vi "3_2_Circular convolution.vi"(4 "N-Point (auto/user def)":enum16{"AUTOMATIC", "USER DEFINED"}(ring), 5 "sequence h[n]":dbl[](array[numeric]), 6 "N-Point":dbl, 7 "sequence x[n]":dbl[](array[numeric])) -> (0 "Sequence y[n] = x[n] * h[n]":dbl[](graph), 1 "Sequence h[n]":dbl[](graph), 2 "Sequence x[n]":dbl[](graph), 3 "sequence y[n] = x[n] * h[n]":dbl[](array[numeric]))   [LabVIEW 2009]
panel:
  in  "stop":bool
  # "CIRCULAR CONVOLUTION"
  # "Program Developed by Indranil Sinharoy"
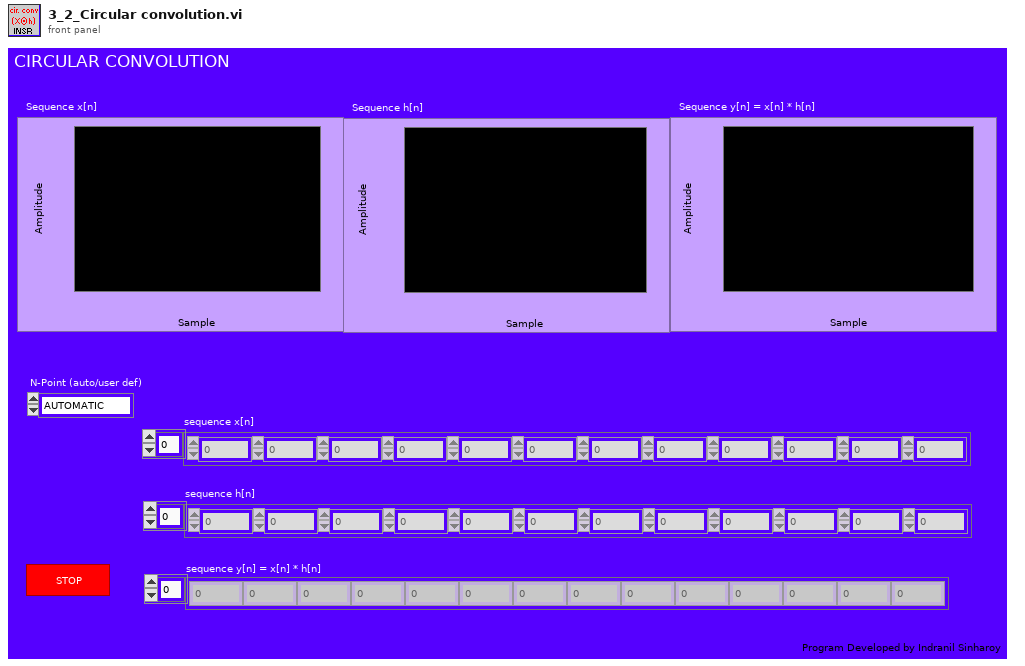
[diagram p1: front panel]
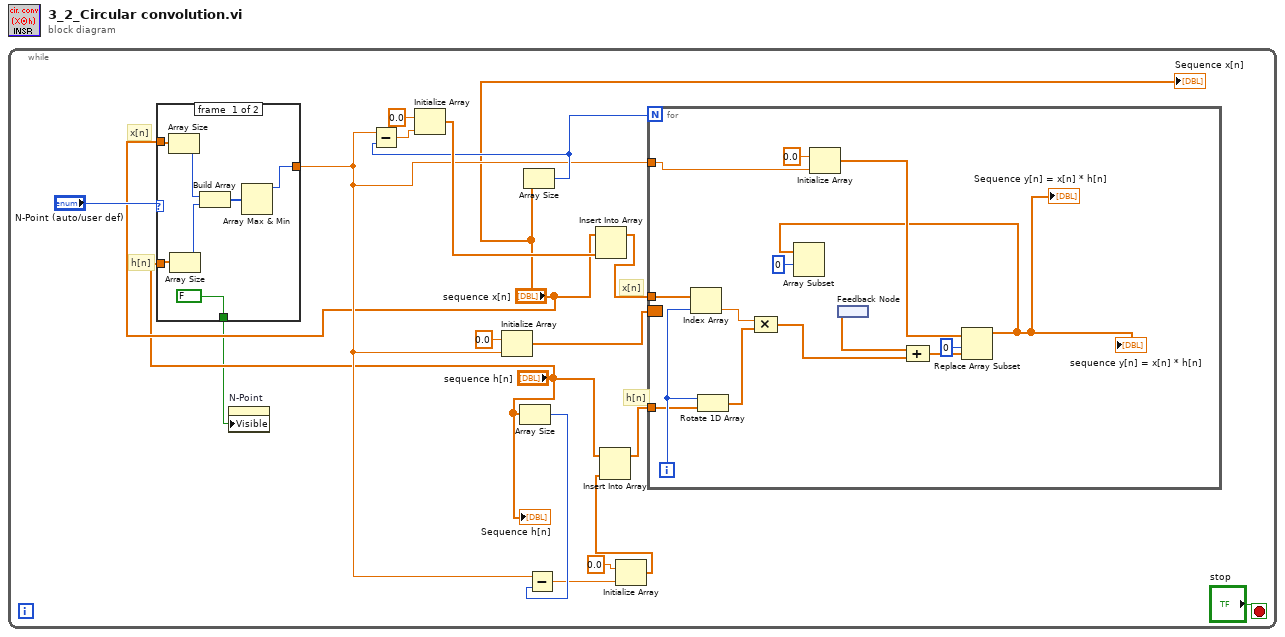
[diagram p0: block diagram]
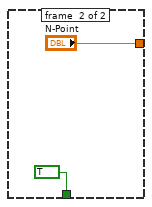
[diagram p2: hidden frame]
diagram:
  n1 = while {
    stop <- "stop" stop-if-true
    # "h[n]"
    # "x[n]"
    # "h[n]"
    # "x[n]"
    n2 = case shown="\"AUTOMATIC\", Default" "N-Point (auto/user def)" {
      tunnel: [w20 "N-Point"] -> w5
      tunnel: "sequence x[n]" -> [w25 _]
      tunnel: "sequence h[n]" -> [w24 _]
      tunnel: [FALSE TRUE] -> w2
      frame #0 {
        n3 = Array Size(array=w25) -> (size(s)=w23:i32)
        n4 = Array Size(array=w24) -> (size(s)=w22:i32)
        n5 = Build Array(w23, w22) -> (w21:i32[])
        n6 = Array Max & Min(array=w21) -> (max value=w20:i32)  [unwired: 3 out]
      }
      frame #1 {
      }
    }
    n7 = property on="N-Point" class="DigNum (strict)"("Visible"=w2) -> ()  [unwired: 2 in, 2 out]
    n8 = Initialize Array "Initialize Array"(0.0 ("element"), w5) -> (w17:dbl[])
    n9 = Array Size(array="sequence h[n]") -> (size(s)=w15:i32)
    n10 = Array Size(array="sequence x[n]") -> (size(s)=w7:i32)
    n11 = Subtract(x=w5, y=w7) -> (x-y=w10:dbl)
    n12 = Initialize Array(0.0 ("element"), w10) -> (w8:dbl[])
    n13 = Subtract(x=w5, y=w15) -> (x-y=w14:dbl)
    n14 = Insert Into Array(array="sequence x[n]", new element=w8) -> (w9:dbl[])  [unwired: 1 in]
    n15 = Initialize Array(0.0 ("element"), w14) -> (w13:dbl[])
    n16 = Insert Into Array(array="sequence h[n]", new element=w13) -> (w11:dbl[])  [unwired: 1 in]
    n17 = for {
      N: w7 -> [_]
      tunnel: w9 -> [w42]
      tunnel: w11 -> [w29]
      tunnel: w5 -> [w28]
      border: w17 -> [_]
      i -> [w30]
      n18 = Index Array "Index Array"(array=w42, index=w30) -> (element=w40:dbl)
      n19 = Rotate 1D Array(1:w29, 2:w30) -> (0:w31:dbl[])
      n20 = Compound Arithmetic op=MULTIPLY(w40, w31) -> (w41:dbl[])
      n21 = Initialize Array "Initialize Array"(0.0 ("element"), w28) -> (w33:dbl[])
      n22 = feedback #1() -> (w37:dbl[])
      n23 = Compound Arithmetic op=ADD(w37, w41) -> (w39:dbl[])
      n24 = Replace Array Subset "Replace Array Subset"(array=w33, new element=w39, index=0) -> (w32:dbl[])
      "sequence y[n] = x[n] * h[n]" <- w32
      "Sequence y[n] = x[n] * h[n]" <- w32
      n25 = Array Subset "Array Subset"(array=w32, index=0) -> (w38:dbl[])  [unwired: 1 in]
    }
    "Sequence x[n]" <- "sequence x[n]"
    "Sequence h[n]" <- "sequence h[n]"
  }
